vi "Do.vi"(8 "error in (no error)":errorcluster, 10 "Actor in":refnum<class "Actor.lvclass">, 11 "RDS Serial Handle Frame Msg in":refnum<class "RDS Serial Handle Frame Msg.lvclass">) -> (0 "error out":errorcluster, 2 "Actor out":refnum<class "Actor.lvclass">)   [LabVIEW 2015, in "RDS Abstracts.lvlib" / "RDS Serial Instrument Actor.lvlib" / "RDS Serial Handle Frame Msg.lvclass"]
doc: "(<B>Filename</B>: Actor Framework.lvlib:Message.lvclass:Do.vi)\n\nDefines what a message does when it is received by an actor. Generally, a message instructs an actor to invoke one of its methods. By default, this method does nothing. A child class must override it to define behavior. Create a child class by using the Actor Framework Message Maker dialog box."
uses:
  RDS Serial Handle Frame Msg.lvclass
  <vilib>/ActorFramework/Actor/Actor.lvclass
  RDS Serial Instrument Actor/RDS Serial Instrument Actor.lvclass
  RDS Serial Handle Frame Msg.lvclass/RDS Serial Handle Frame Msg.ctl
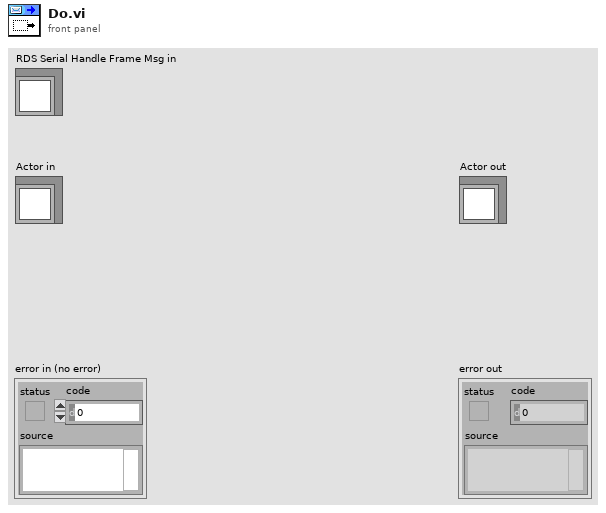
[diagram p1: front panel]
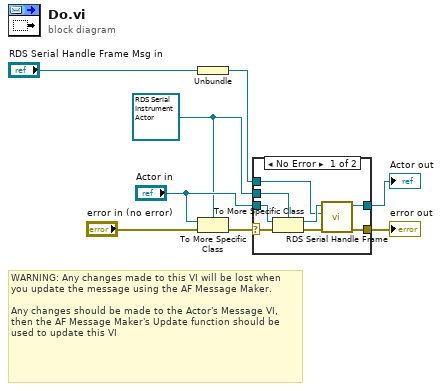
[diagram p0: block diagram]
diagram:
  w3 = refnum<class "RDS Serial Instrument Actor.lvclass"> refnum ("Actor Type")
  # "WARNING: Any changes made to this VI will be lost when you update the message using the AF Message Maker.\n\nAny changes should be made to the Actor's Message VI, then the AF Message Maker's Update function should be used to update this VI"
  n1 = Unbundle("RDS Serial Handle Frame Msg in") -> (w2:refnum<class "RDS Serial Frame.lvclass">)
  n2 = To More Specific Class(target class=w3, reference="Actor in", error in="error in (no error)") -> (error out=w7:errorcluster)  [unwired: 1 out]
  n3 = case shown="No Error" w7 {
    selector: w7 -> [w16 w18]
    tunnel: [w11 w18] -> w6
    tunnel: [w10 w17] -> w5
    tunnel: "Actor in" -> [w15 w17]
    tunnel: w3 -> [w14 _]
    tunnel: w2 -> [w9 _]
    frame No Error {
      n4 = To More Specific Class ("Actor Cast")(target class=w14, reference=w15, error in=w16) -> (specific class reference=w13:refnum<class "RDS Serial Instrument Actor.lvclass">, error out=w12:errorcluster)
      n5 = call-dynamic "RDS Serial Handle Frame.vi"("error in (no error)"=w12, "RDS Serial Frame"=w9, "RDS Serial Instrument Actor in"=w13) -> ("error out"=w11:errorcluster, "RDS Serial Instrument Actor out"=w10:refnum<class "RDS Serial Instrument Actor.lvclass">)  [unwired: 7 in]
    }
    frame Error {
    }
  }
  "error out" <- w6
  "Actor out" <- w5
